vi "Queue Init.vi"(8 "error in (no error)":errorcluster, 11 "Father of all uServices in":refnum<class "Father of all uServices.lvclass">) -> (0 "error out":errorcluster, 3 "Father of all uServices out":refnum<class "Father of all uServices.lvclass">)   [LabVIEW 2026, in "TALOS.lvlib" / "Father of all uServices.lvlib" / "Father of all uServices.lvclass"]
uses:
  Father of all uServices.lvclass
  Msg to uServ Selector.ctl
  Event Handler Items.ctl
  Father of all uServices.lvclass/Father of all uServices.ctl
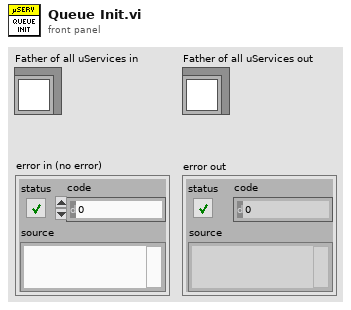
[diagram p1: front panel]
types:
  T1 = typedef "TALOS.lvlib/Father of all uServices.lvlib/Father of all uServices.lvclass/Event Handler Items.ctl" = enum16{"Button Pressed", "Message", "Ready to launch?", "Safe Mode", "Start RUN", "Stop RUN"}
  T2 = cluster{"Event Item":T1, "Event Item Name":string, "Event Data":variant}
  T3 = typedef "TALOS.lvlib/Father of all uServices.lvlib/Father of all uServices.lvclass/Msg to uServ Selector.ctl" = enum16{"Test string"}
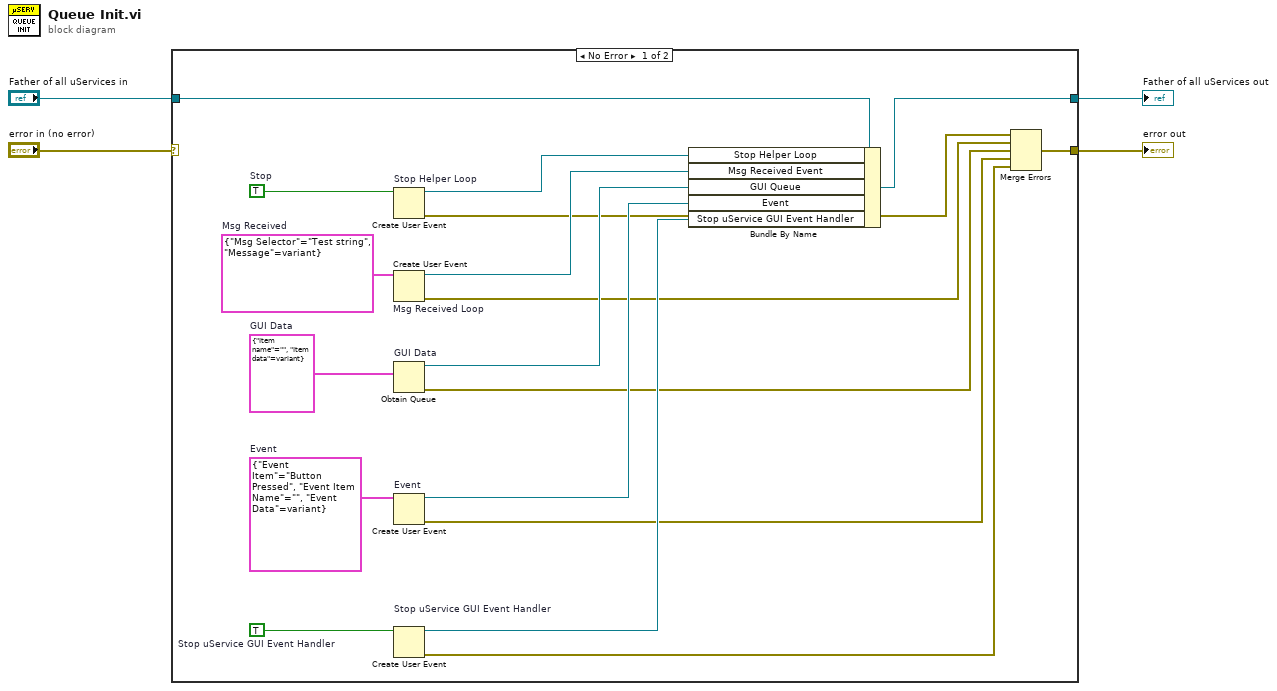
[diagram p0: block diagram]
diagram:
  n1 = case shown="No Error" "error in (no error)" {
    selector: "error in (no error)" -> [_ w24]
    tunnel: "Father of all uServices in" -> [w5 w23]
    tunnel: [w10 w23] -> w3
    tunnel: [w9 w24] -> w2
    frame No Error {
      w20 = TRUE  # Stop uService GUI Event Handler
      w17 = T2 {"Event Item"=enum."Button Pressed", "Event Item Name"="", "Event Data"=variant}  # Event
      w14 = cluster{"Item name":string, "Item data":variant} {"Item name"="", "Item data"=variant}  # GUI Data
      w12 = cluster{"Msg Selector":T3, "Message":variant} {"Msg Selector"=enum."Test string", "Message"=variant}  # Msg Received
      w6 = TRUE  # Stop
      n2 = Create User Event "Stop Helper Loop"(user event datatype=w6) -> (user event=w7:refnum<user-event>, error out=w8:errorcluster)  [unwired: 1 in]
      n3 = Create User Event "Msg Received Loop"(user event datatype=w12) -> (user event=w13:refnum<user-event>, error out=w11:errorcluster)  [unwired: 1 in]
      n4 = Obtain Queue "GUI Data"(element data type=w14) -> (queue out=w16:refnum<queue>, error out=w15:errorcluster)  [unwired: 4 in, 1 out]
      n5 = Create User Event "Event"(user event datatype=w17) -> (user event=w19:refnum<user-event>, error out=w18:errorcluster)  [unwired: 1 in]
      n6 = Create User Event "Stop uService GUI Event Handler"(user event datatype=w20) -> (user event=w22:refnum<user-event>, error out=w21:errorcluster)  [unwired: 1 in]
      n7 = Bundle By Name(cluster=w5, "Stop Helper Loop"=w7, "Msg Received Event"=w13, "GUI Queue"=w16, "Event"=w19, "Stop uService GUI Event Handler"=w22) -> (w10:refnum<class "Father of all uServices.lvclass">)
      n8 = Merge Errors(w8, w11, w15, w18, w21) -> (w9:errorcluster)
    }
    frame Error {
    }
  }
  "Father of all uServices out" <- w3
  "error out" <- w2
